vi "ClearReference.vi"(1 "reference in":refnum<class "G#Interface.lvclass">) -> (0 "reference out":refnum<class "G#Interface.lvclass">)   [LabVIEW 2020, in "G#Interface.lvclass"]
doc: "Clears the object reference and makes it invalid.\n\nNotice, this will not delete the object!"
uses:
  G#Interface.lvclass
  G#Interface.lvclass/G#Interface.ctl
  G#Object/G#Object.lvclass
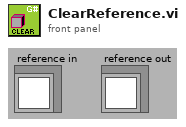
[diagram p1: front panel]
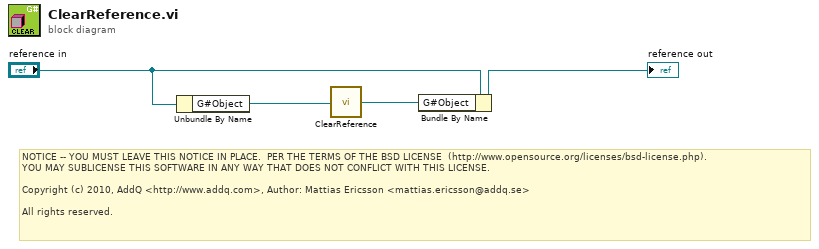
[diagram p0: block diagram]
diagram:
  # "NOTICE -- YOU MUST LEAVE THIS NOTICE IN PLACE.  PER THE TERMS OF THE BSD LICENSE  (http://www.opensource.org/licenses/bsd-license.php).\nYOU MAY SUBLICENSE THIS SOFTWARE IN ANY WAY THAT DOES NOT CONFLICT WITH THIS LICENSE.\n\nCopyright (c) 2010, AddQ <http://www.addq.com>, Author: Mattias Ericsson <mattias.ericsson@addq.se>\n\nAll rights reserved."
  n1 = Unbundle By Name("reference in") -> ("G#Object"=w4:refnum<class "G#Object.lvclass">)
  n2 = call-dynamic "ClearReference.vi"("reference in"=w4) -> ("reference out"=w2:refnum<class "G#Object.lvclass">)
  n3 = Bundle By Name(cluster="reference in", "G#Object"=w2) -> (→"reference out":refnum<class "G#Interface.lvclass">)
